vi "Initialize Settings.vi"(8 "error in (no error)":errorcluster, 11 "Output Sequencer in":refnum<class "Output Sequencer.lvclass">) -> (0 "error out":errorcluster, 3 "Output Sequencer out":refnum<class "Output Sequencer.lvclass">)   [LabVIEW 2024, in "Output Sequencer.lvlib" / "Output Sequencer.lvclass"]
uses:
  Output Sequencer.lvclass
  C:/Program Files/National Instruments/LabVIEW 2024/vi.lib/FlexLogger/SDK/PluginSDK.lvlibp/PEFClasses/SDK/Plugin/Plugin.lvclass
  Types/UI Event.ctl
  Types/Event Type.ctl
  Types/UI Ref.ctl
  Types/State.ctl
  Types/Sequencer State.ctl
  Output Sequencer.lvclass/Output Sequencer.ctl
  Globals/Global Strings.vi
  <vilib>/FlexLogger/SDK/PluginSDK.lvlibp/PEFClasses/SDK/Plugin/ParameterAccess/Read String.vi
  <vilib>/FlexLogger/SDK/PluginSDK.lvlibp/PEFClasses/SDK/Plugin/ParameterAccess/Write String.vi
  Settings UI/Settings UI.vi
  <vilib>/FlexLogger/SDK/PluginSDK.lvlibp/PEFClasses/SDK/Plugin/Plugin.lvclass
  Settings UI/Settings UI.lvclass
  C:/Program Files/National Instruments/LabVIEW 2024/vi.lib/FlexLogger/SDK/PluginSDK.lvlibp/PEFClasses/SDK/Processing Element/Processing Element.lvclass
  C:/Dev/GitHub/ni/niflexlogger-plugins/PDK plugins/Output Sequencer/source/Output Sequencer/Output Sequencer.lvclass
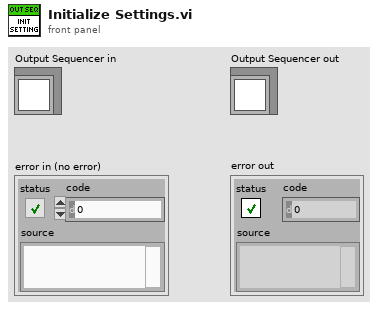
[diagram p1: front panel]
types:
  T1 = typedef "Output Sequencer.lvlib/Output Sequencer.lvclass/UI Ref.ctl" = refnum<vi>
  T2 = typedef "Output Sequencer.lvlib/Output Sequencer.lvclass/UI Event.ctl" = cluster{"Type":T3, "Data":variant}
  T3 = typedef "Output Sequencer.lvlib/Output Sequencer.lvclass/Event Type.ctl" = enum16{"Channel Update", "Test State Change", "Stop"}
  T4 = typedef "Output Sequencer.lvlib/Settings UI.lvclass/Settings.ctl" = cluster{"Plug-in Version":string, "Step Values":T5[], "Only Execute When Test Running":bool, "Reset Sequence When Test Starts":bool, "Number of Sequence Steps":i32, "Num of Analog Channels":i32, "Num of Digital Channels":i32, "Delay Before Starting Sequence":dbl, "Default Analog Values":dbl[], "Default Digital Values":bool[], "Max Iterations":u32, "Use last value when stopped":bool, "Prioritize exact values":bool, "Enable advanced step timing":bool, "Enable step conditions":bool, "Show confirmation dialogs":bool, "Start condition":string, "Enable re-triggering":bool, "Stop condition":string}
  T5 = typedef "Output Sequencer.lvlib/Settings UI.lvclass/Step Settings.ctl" = cluster{"Description":string, "Precondition":string, "Duration":dbl, "Mode":string, "Delay Between Values":dbl, "Analog Values":string[], "Digital Values":string[], "Postcondition":string, "On True":string, "On False":string}
  T6 = typedef "Output Sequencer.lvlib/Output Sequencer.lvclass/State.ctl" = cluster{"Configured":bool, "Reconfigure Pending":bool, "Current Step":i32, "Total Iterations":i32, "Current Step Start Timestamp":dbl, "Time Remaining":dbl, "Test Running":bool, "Pause Timestamp":dbl, "Last Output Analog Values":dbl[], "Last Output Digital Values":bool[], "Previous Step Analog Values":dbl[], "Previous Step Digital Values":bool[], "Sequencer State":T7}
  T7 = typedef "Output Sequencer.lvlib/Output Sequencer.lvclass/Sequencer State.ctl" = enum16{"Error", "Initialize", "Prepare channels", "Wait for test", "Wait for %.1f sec", "Wait for trigger", "Stop condition", "Wait for resume", "Running", "Paused", "No valid step", "Stopped"}
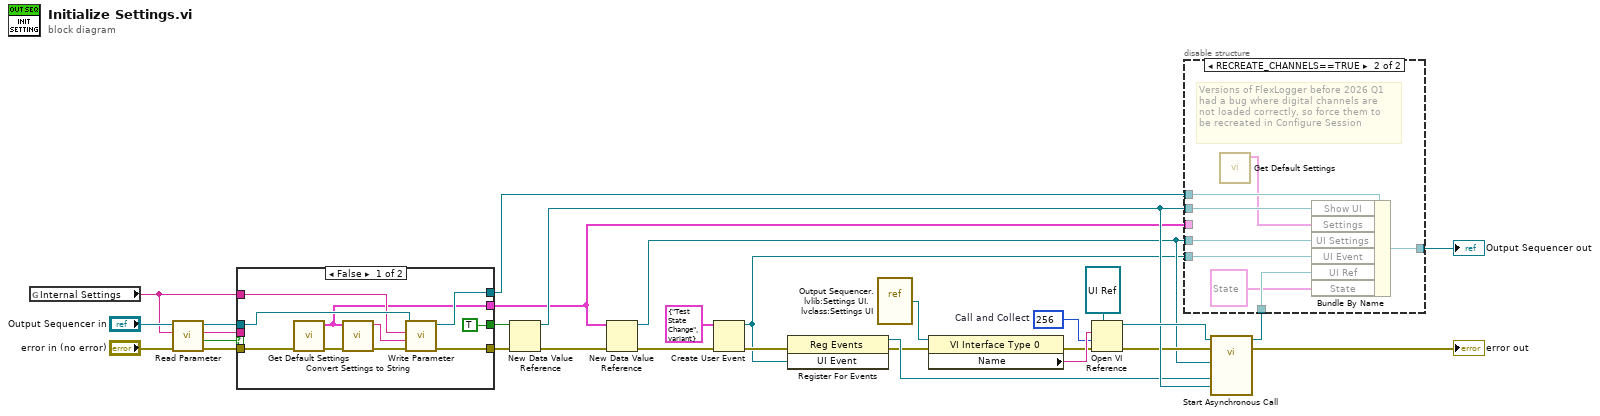
[diagram p0: block diagram]
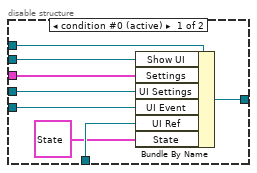
[diagram p2: hidden frame]
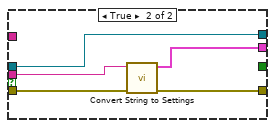
[diagram p3: hidden frame]
diagram:
  w17 = 256  # Call and Collect
  n1 = global read "Global Strings.vi" "Internal Settings"() -> (w24:string)
  n2 = call-poly <vilib>:"Read Parameter.vi"("error in (no error)"="error in (no error)", "Name"=w24, "Plugin in"="Output Sequencer in") -> ("error out"=w25:errorcluster, "Found"=w14:bool, "Value"=w23:string, "Plugin out"=w26:refnum<class "Output Sequencer.lvclass">)  [unwired: 5 in]
  n3 = case shown="False" w14 {
    tunnel: [w39 w41] -> w7
    tunnel: [w38 w45] -> w12
    tunnel: w26 -> [w37 w45]
    tunnel: w25 -> [w34 w42]
    tunnel: w24 -> [w36 _]
    tunnel: w23 -> [_ w44]
    tunnel: [w35 w43] -> w13
    tunnel: [TRUE _] -> w1
    frame False {
      n4 = call "Get Default Settings.vi"("error in (no error)"=w34) -> ("error out"=w33:errorcluster, "Settings out"=w35:T4)  [unwired: 9 in]
      n5 = call "Convert Settings to String.vi"("error in (no error)"=w33, "Settings in"=w35) -> ("error out"=w32:errorcluster, "String out"=w40:string)  [unwired: 8 in]
      n6 = call-poly <vilib>:"Write Parameter.vi"("error in (no error)"=w32, "Value"=w40, "Name"=w36, "Plugin in"=w37) -> ("error out"=w39:errorcluster, "Plugin out"=w38:refnum<class "Output Sequencer.lvclass">)  [unwired: 6 in]
    }
    frame True {
      n7 = call "Convert String to Settings.vi"("error in (no error)"=w42, "String In"=w44) -> ("error out"=w41:errorcluster, "Settings Out"=w43:T4)  [unwired: 8 in]
    }
  }
  n8 = New Data Value Reference(data value=w1, error in=w7) -> (data value reference=w21:refnum<data-value>, error out=w6:errorcluster)
  n9 = New Data Value Reference(data value=w13, error in=w6) -> (data value reference=w3:refnum<data-value>, error out=w5:errorcluster)
  n10 = Create User Event(user event datatype=T2 {"Type"=enum."Test State Change", "Data"=variant} ("UI Event"), error in=w5) -> (user event=w2:refnum<user-event>, error out=w9:errorcluster)
  n11 = register-events(error in=w9, w2) -> (reference out=w19:refnum<event-registration>, error out=w8:errorcluster)  [unwired: 1 in]
  n12 = vi-ref "Output Sequencer.lvlib:Settings UI.lvclass:Settings UI.vi"() -> (w15:refnum<vi>)
  n13 = property class="VI Interface Type 0"(reference=w15, error in=w8) -> (error out=w11:errorcluster, "Name"=w18:string)  [unwired: 1 out]
  n14 = Open VI Reference(type specifier VI Refnum (for type only)=T1 refnum ("Cust UI"), vi path=w18, options=w17, error in (no error)=w11) -> (vi reference=w22:T1, error out=w10:errorcluster)  [unwired: 2 in]
  n15 = call-by-ref "Start Asynchronous Call"(reference=w22, error in=w10, "Show UI"=w21, "UI Event Registration"=w19, "Applied Settings"=w3) -> (reference out=w4:T1, error out=→"error out":errorcluster)  [unwired: 9 in]
  n16 = disable-structure shown="RECREATE_CHANNELS==TRUE" {
    disable-tunnel: [w53 w61] -> w30
    disable-tunnel: w21 -> [w52 w60]
    disable-tunnel: w13 -> [w51 _]
    disable-tunnel: w12 -> [w50 w59]
    disable-tunnel: w4 -> [w49 w58]
    disable-tunnel: w3 -> [w48 w57]
    disable-tunnel: w2 -> [w47 w56]
    frame condition #0 (active) {
      n17 = Bundle By Name(cluster=w50, "Show UI"=w52, "Settings"=w51, "UI Settings"=w48, "UI Event"=w47, "UI Ref"=w49, "State"=T6 {"Configured"=FALSE, "Reconfigure Pending"=FALSE, "Current Step"=0, "Total Iterations"=0, "Current Step Start Timestamp"=0.0, "Time Remaining"=0.0, "Test Running"=FALSE, "Pause Timestamp"=0.0, "Last Output Analog Values"=[], "Last Output Digital Values"=[], "Previous Step Analog Values"=[], "Previous Step Digital Values"=[], "Sequencer State"=enum."Initialize"}) -> (w53:refnum<class "Output Sequencer.lvclass">)
    }
    frame condition #1 {
      # "Versions of FlexLogger before 2026 Q1\nhad a bug where digital channels are\nnot loaded correctly, so force them to\nbe recreated in Configure Session"
      n18 = call "Get Default Settings.vi"() -> ("Settings out"=w54:T4)  [unwired: 10 in, 1 out]
      n19 = Bundle By Name(cluster=w59, "Show UI"=w60, "Settings"=w54, "UI Settings"=w57, "UI Event"=w56, "UI Ref"=w58, "State"=T6 {"Configured"=FALSE, "Reconfigure Pending"=FALSE, "Current Step"=0, "Total Iterations"=0, "Current Step Start Timestamp"=0.0, "Time Remaining"=0.0, "Test Running"=FALSE, "Pause Timestamp"=0.0, "Last Output Analog Values"=[], "Last Output Digital Values"=[], "Previous Step Analog Values"=[], "Previous Step Digital Values"=[], "Sequencer State"=enum."Initialize"}) -> (w61:refnum<class "Output Sequencer.lvclass">)
    }
  }
  "Output Sequencer out" <- w30
